vi "recalculate galvo waveform.vi"(8 "error in (no error)":errorcluster, 11 "Waveform in":refnum<class "Waveform.lvclass">) -> (0 "error out":errorcluster, 3 "Waveform out":refnum<class "Waveform.lvclass">)   [LabVIEW 2012, in "Waveform.lvclass"]
uses:
  Waveform.lvclass
  Waveform.lvclass/Waveform.ctl
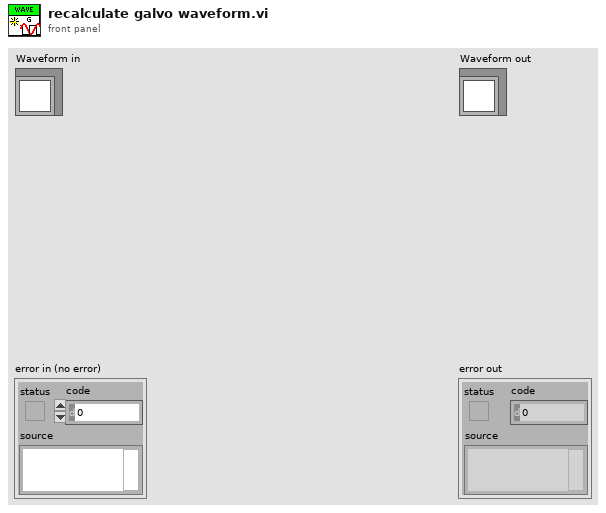
[diagram p1: front panel]
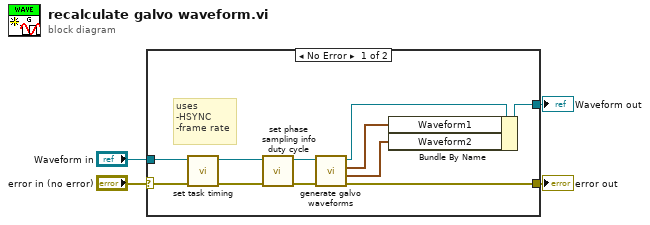
[diagram p0: block diagram]
diagram:
  n1 = case shown="No Error" "error in (no error)" {
    selector: "error in (no error)" -> [w13 w17]
    tunnel: [w9 w17] -> w3
    tunnel: [w7 w16] -> w1
    tunnel: "Waveform in" -> [w12 w16]
    frame No Error {
      # "uses \n-HSYNC\n-frame rate"
      n2 = call-dynamic "set task timing.vi"("error in (no error)"=w13, "Waveform in"=w12) -> ("error out"=w11:errorcluster, "Waveform out"=w10:refnum<class "Waveform.lvclass">)  [unwired: 8 in]
      n3 = call-dynamic "set phase sampling info duty cycle.vi"("error in (no error)"=w11, "Waveform in"=w10) -> ("error out"=w15:errorcluster, "Waveform out"=w14:refnum<class "Waveform.lvclass">)  [unwired: 8 in]
      n4 = call-dynamic "generate galvo waveforms.vi"("error in (no error)"=w15, "Waveform in"=w14) -> ("error out"=w9:errorcluster, "Waveform 2"=w5:waveform(dbl), "Waveform"=w6:waveform(dbl), "Waveform out"=w8:refnum<class "Waveform.lvclass">)  [unwired: 6 in]
      n5 = Bundle By Name(cluster=w8, "Waveform1"=w6, "Waveform2"=w5) -> (w7:refnum<class "Waveform.lvclass">)
    }
    frame Error {
    }
  }
  "error out" <- w3
  "Waveform out" <- w1
